vi "Approach then CV VUW.vi"(7 "Computer called (T/F)":bool) -> ()   [LabVIEW 2023]
uses:
  Sub_Vi/TypeDefsControls/Zposition.ctl
  Sub_Vi/TypeDefsControls/Piezo Velocity.ctl
  Sub_Vi/TypeDefsControls/Voltage.ctl
  Sub_Vi/TypeDefsControls/Xposition.ctl
  Sub_Vi/TypeDefsControls/Yposition.ctl
  Sub_Vi/TypeDefsControls/Voltage Scan Rate.ctl
  Sub_Vi/TypeDefsControls/Iterator.ctl
  Sub_Vi/TypeDefs/WayPointCluster.ctl
  Sub_Vi/TypeDefs/ChangeOnFly.ctl
  Sub_Vi/TypeDefs/Settings.ctl
  Sub_Vi/TypeDefs/Display.ctl
  Sub_Vi/TypeDefsControls/Feedback Type.ctl
  Settings.vi
panel:
  in  "Approach Type":u16=2
  out "Current 1":cluster{"Y":dbl[], "Y":dbl[]}[](graph)
  in  "Boolean Negative":bool
  in  "Boolean Positive":bool=TRUE
  in  "Feedback Threshold (A)\nGreater Than":dbl
  in  "Feedback Type":T1=enum."Current 1"
  in  "Display Cluster":T2
  in  "SettingsCluster":T3={"Sample Rate (us)"=1, "Samples Per Data Point (int, power of 2)"=1000, "DistanceToBulk (um)"=-1.0, "HoldTimeScaler"=1, "SaveData"=TRUE, "DistanceToBulk (um) 2"=-1.0, "DistanceToBulk (um) 3"=-1.0}
  in  "ChangeonFly":T4
  in  "WayPointCluster":T5
  in  "Number of Cycles":T6=1.0 min=1.0
  in  "Start scan Button":bool
  in  "Stop":bool
  in  "Pause":bool
  in  "Feedback Threshold (A)\nLess Than":dbl
  in  "Scan Rate (V/s)":T7 min=0.0 max=1000.0
  in  "Second Voltage (V)":T8 min=-10.0 max=10.0
  in  "First Voltage (V)":T8 min=-10.0 max=10.0
  in  "Set X":bool
  in  "Set Y":bool
  in  "Y":T9=100.0 min=0.0 max=100000.0
  in  "X":T10=100.0 min=0.0 max=100000.0
  in  "Approach Voltage (V)":T8 min=-10.0 max=10.0
  in  "Approach Rate (µm/s)":T11=0.1 min=0.0
  in  "End Extension (µm)":T12 min=0.0 max=100000.0
  in  "Start Extention (µm)":T12=150.0 min=0.0 max=100000.0
  out "?":cluster{"Y":dbl[], "Y":dbl[]}[](graph)
  out "?":dbl[](graph)
  # "Settings"
  # "Pause at"
  # "Advanced Settings"
  # "CV Controls"
  # "Voltage Profile"
  # "Approach"
  # "First Cycle"
  # "Additional Cycles"
  # "Retract"
  # "First\nVoltage"
  # "Approach\nVoltage"
  # "(Number of \ncycles)"
  # "Second\nVoltage"
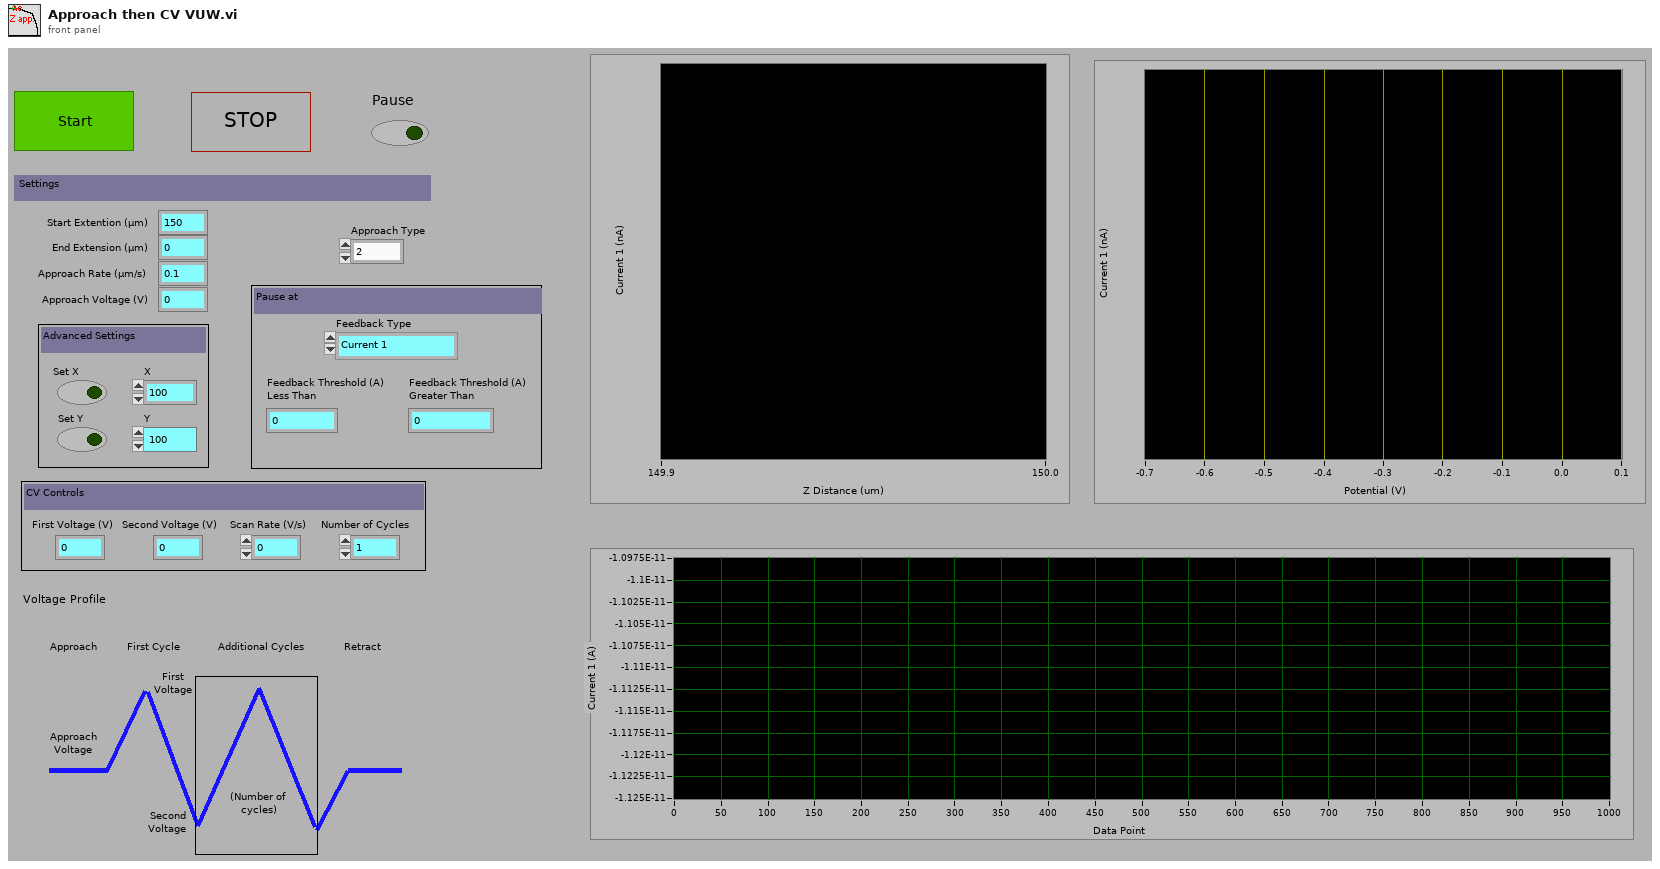
[diagram p1: front panel]
types:
  T1 = typedef "Feedback Type.ctl" = enum16{"AC Magnitude", "Current 1", "Current 2", "Phase"}
  T2 = typedef "Display.ctl" = cluster{"X":refnum<vi>, "Y":refnum<vi>, "Z":refnum<vi>, "Amp":refnum<vi>, "Phase":refnum<vi>, "t vs Z":refnum<vi>, "t vs C1":refnum<vi>, "t vs C2":refnum<vi>, "t vs C3":refnum<vi>, "t vs Amp":refnum<vi>, "t vs Phase":refnum<vi>, "t vs X":refnum<vi>, "t vs Y":refnum<vi>, "Z vs C1":refnum<vi>, "Z vs C2":refnum<vi>, "Z vs C3":refnum<vi>, "V vs C1":refnum<vi>, "V vs C2":refnum<vi>, "V vs C3":refnum<vi>, "X/Y/Z F":refnum<vi>, "X/Y/Z R":refnum<vi>, "X/Y/C1 F":refnum<vi>, "X/Y/C1 R":refnum<vi>, "X/Y/C2 F":refnum<vi>, "X/Y/C2 R":refnum<vi>, "X/Y/C3 F":refnum<vi>, "X/Y/C3 R":refnum<vi>, "NumberOfLines":u16, "um Per Pixel":dbl, "um Per Line":dbl, "X Center":dbl, "Hop X/Y/Z":refnum<vi>, "Hop X/Y/C1":refnum<vi>, "Hop X/Y/C2":refnum<vi>, "Hop X/Y/C3":refnum<vi>, "X Width":dbl, "Y Width":dbl, "Hopping Distance":dbl, "V2 vs C1":refnum<vi>, "V vs Phase":refnum<vi>, "Y Center":dbl, "Number of Pixels":dbl, "V2 vs C2":refnum<vi>, "V2 vs C3":refnum<vi>, "V vs y":refnum<vi>, "V2 vs y":refnum<vi>, "Z vs Amp":refnum<vi>, "Z vs Phase":refnum<vi>}
  T3 = typedef "Settings.ctl" = cluster{"Sample Rate (us)":u32, "Samples Per Data Point (int, power of 2)":i16, "DistanceToBulk (um)":dbl, "HoldTimeScaler":u64, "SaveData":bool, "DistanceToBulk (um) 2":dbl, "DistanceToBulk (um) 3":dbl}
  T4 = typedef "ChangeOnFly.ctl" = cluster{"Stop (boolean)":refnum<vi>, "Pause (boolean)":refnum<vi>, "EndCurrentLine (boolean)":refnum<vi>, "max movement per update step (Interger, nm)":refnum<vi>, "P (float, arb)":refnum<vi>, "Feedback set point (double, Amps)":refnum<vi>, "Voltage (double, V)":refnum<vi>, "Feedback set point 2 (double, Amps)":refnum<vi>, "Stop on Greater Than 2? (boolean)":refnum<vi>, "Stop on Greater Than? (boolean)":refnum<vi>, "Voltage 2 (double, V)":refnum<vi>, "Feedback Type (enum)":refnum<vi>, "Feedback Type 2 (enum)":refnum<vi>}
  T5 = typedef "WayPointCluster.ctl" = cluster{"X (um)":dbl[], "Y (um)":dbl[], "Z (um)":dbl[], "V (V)":dbl[], "X Velocity (um s-1)":dbl[], "Y Velocity (um s-1)":dbl[], "Z Velocity (um s-1)":dbl[], "V Velocity (V s-1)":dbl[], "FeedBack Type (enum)":u16[], "Move X (boolean)":bool[], "Move Y (boolean)":bool[], "Move Z (boolean)":bool[], "Move V (boolean)":bool[], "Jump V (boolean)":bool[], "Hold (boolean)":bool[], "Hold Time":u32[], "V2 (V)":dbl[], "Move V2":bool[], "V2 Velocity (V s-1)":dbl[], "Jump V2 (boolean)":bool[], "Update z Position delta (ms)":i16[], "Hold Feedback1":bool[], "Move Z PicoMotor":bool[], " Z PicoMotor Direction":bool[], "DIO0":bool[]}
  T6 = typedef "Iterator.ctl" = dbl
  T7 = typedef "Voltage Scan Rate.ctl" = dbl
  T8 = typedef "Voltage.ctl" = dbl
  T9 = typedef "Yposition.ctl" = dbl
  T10 = typedef "Xposition.ctl" = dbl
  T11 = typedef "Piezo Velocity.ctl" = dbl
  T12 = typedef "Zposition.ctl" = dbl
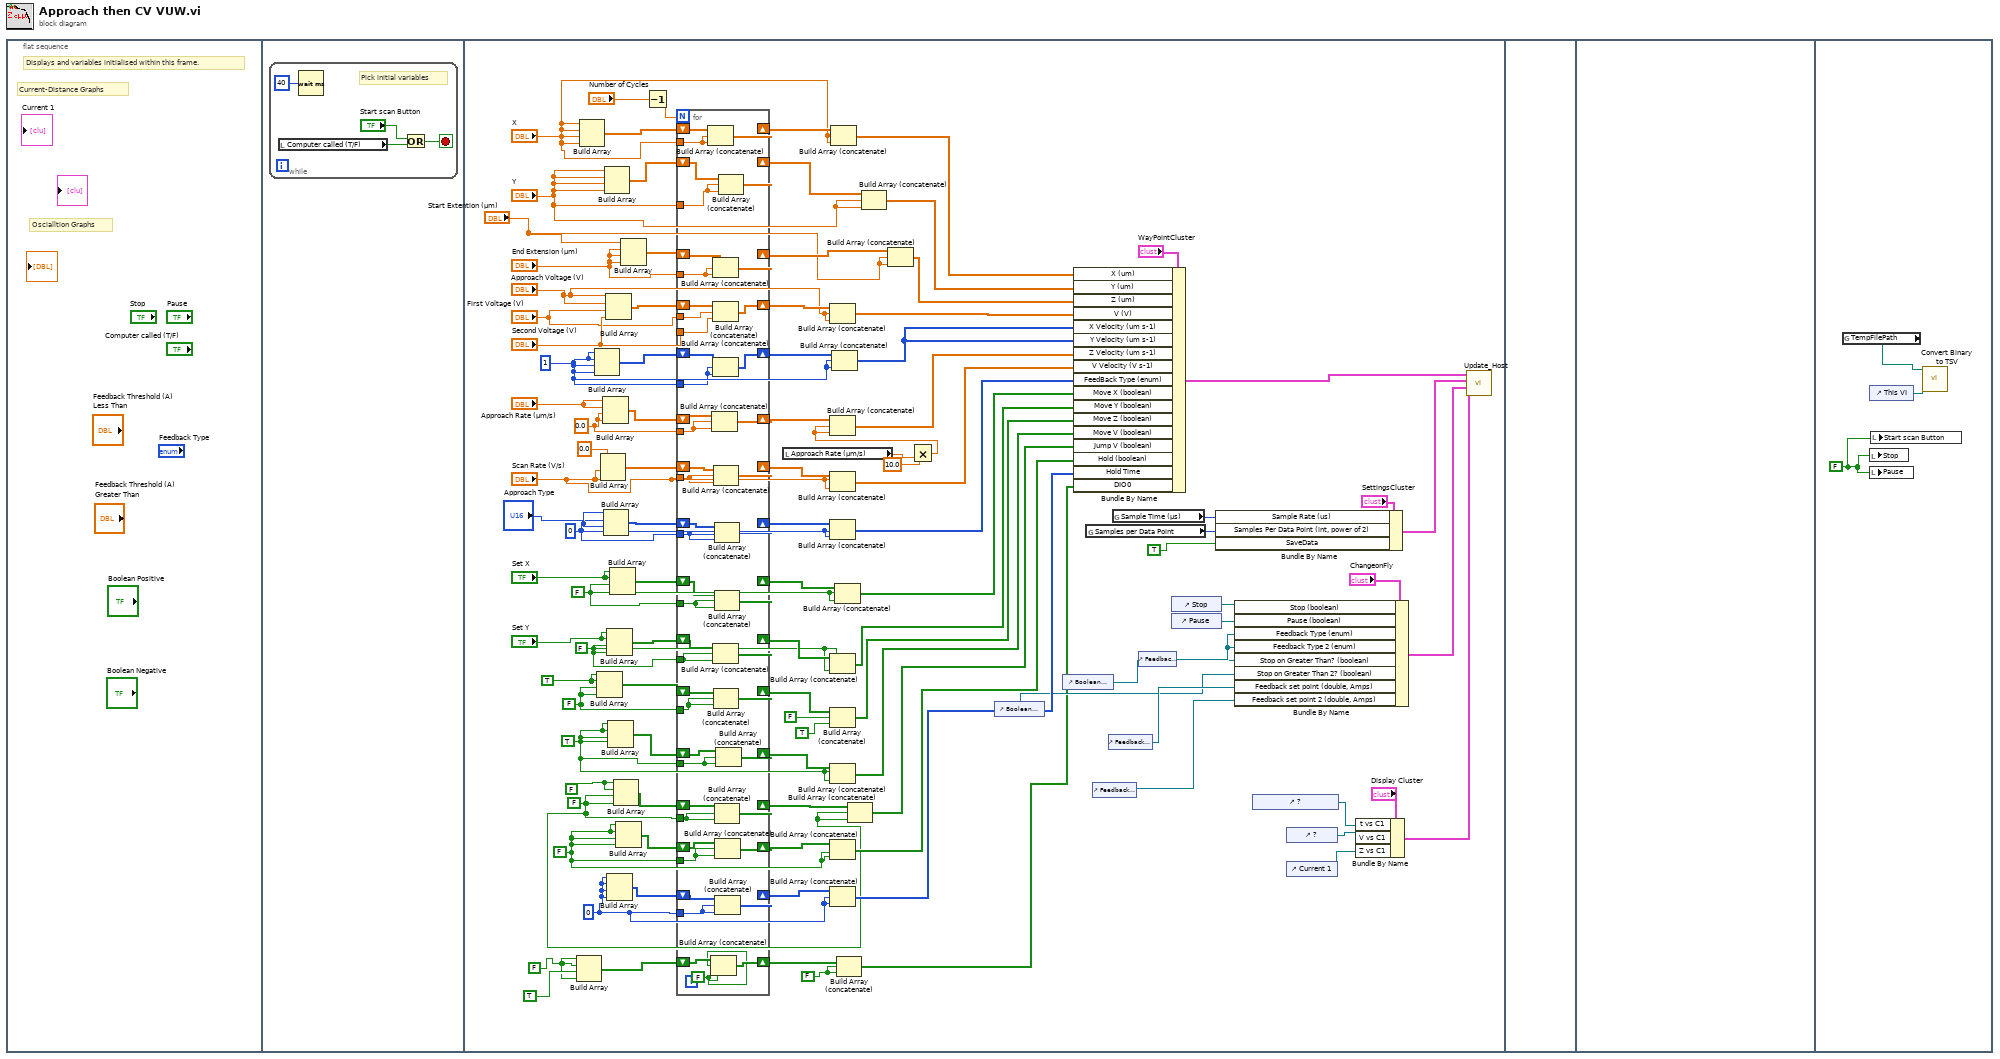
[diagram p0: block diagram]
diagram:
  n1 = flat-sequence {
    frame #0 {
      # "Oscialltion Graphs"
      # "Current-Distance Graphs"
      # "Displays and variables initialised within this frame."
    }
    frame #1 {
      n2 = while {
        stop <- w4 stop-if-true
        # "Pick initial variables"
        n3 = local read "Computer called (T/F)"() -> (w2:bool)
        n4 = Wait (ms)(milliseconds to wait=u32 40) -> ()  [unwired: 1 out]
        n5 = Or(x="Start scan Button", y=w2) -> (x .or. y?=w4:bool)
      }
    }
    frame #2 {
      w12 = FALSE ("Set Z")
      w6 = FALSE ("Set Z")
      w25 = u32 0 ("element")
      w9 = FALSE ("element")
      w8 = FALSE ("Set Z")
      w27 = TRUE ("element")
      w89 = FALSE ("element")
      w29 = FALSE ("element")
      w28 = FALSE ("element")
      w30 = u16 0 ("element")
      w54 = 0.0
      w34 = 0.0 ("element")
      w26 = FALSE ("Set Z")
      w51 = TRUE ("Set Z")
      w35 = 1
      n6 = Build Array(w6, w6, TRUE ("Set Z"), w6) -> (w14:bool[])
      n7 = Build Array("X", "X", "X", "X") -> (w59:T10[])
      n8 = Build Array(w35, w35, w35, w35) -> (w74:i32[])
      n9 = Build Array(w51, w51, w89, w89) -> (w90:bool[])
      n10 = Build Array(w54, w54, "Scan Rate (V/s)", "Scan Rate (V/s)") -> (w79:T7[])
      n11 = Build Array("Approach Rate (µm/s)", "Approach Rate (µm/s)", w34, w34) -> (w77:T11[])
      n12 = Build Array(w30, "Approach Type", w30, w30) -> (w82:u16[])
      n13 = Build Array("Y", "Y", "Y", "Y") -> (w62:T9[])
      n14 = Build Array("Approach Voltage (V)", "Approach Voltage (V)", "First Voltage (V)", "Second Voltage (V)") -> (w101:T8[])
      n15 = Build Array("Set Y", "Set Y", w28, w28) -> (w87:bool[])
      n16 = Build Array(w25, w25, w25, w25) -> (w100:u32[])
      n17 = Build Array(w27, w27, w27, w27) -> (w92:bool[])
      n18 = Build Array("Set X", "Set X", w29, w29) -> (w85:bool[])
      n19 = Build Array(w8, w8, w9, w9) -> (w94:bool[])
      n20 = Build Array(w26, w26, w26, w26) -> (w97:bool[])
      n21 = Build Array("Start Extention (µm)", "End Extension (µm)", "End Extension (µm)", "End Extension (µm)") -> (w41:T12[])
      n22 = Decrement(x="Number of Cycles") -> (x-1=w40:T6)
      n23 = for {
        N: w40 -> [_]
        tunnel: "First Voltage (V)" -> [w155]
        shift-right: [w156] -> w103
        shift-left: w101 -> [w157]
        tunnel: "Second Voltage (V)" -> [w154]
        shift-right: [w152] -> w99
        shift-left: w100 -> [w153]
        tunnel: w25 -> [w151]
        shift-right: [w148] -> w96
        shift-left: w97 -> [w149]
        tunnel: w26 -> [w150]
        shift-right: [w145] -> w93
        shift-left: w94 -> [w147]
        tunnel: w9 -> [w146]
        shift-right: [w143] -> w83
        shift-left: w92 -> [w144]
        tunnel: w27 -> [w142]
        shift-right: [w140] -> w91
        shift-left: w90 -> [w141]
        tunnel: w89 -> [w139]
        shift-right: [w137] -> w88
        shift-left: w87 -> [w138]
        tunnel: w28 -> [w136]
        shift-right: [w135] -> w84
        shift-left: w85 -> [w134]
        tunnel: w29 -> [w133]
        shift-right: [w131] -> w81
        shift-left: w82 -> [w132]
        tunnel: w30 -> [w130]
        shift-right: [w128] -> w80
        shift-left: w79 -> [w129]
        tunnel: "Scan Rate (V/s)" -> [w127]
        shift-right: [w125] -> w78
        shift-left: w77 -> [w126]
        tunnel: w34 -> [w124]
        shift-right: [w122] -> w75
        shift-left: w74 -> [w123]
        tunnel: w35 -> [w121]
        shift-right: [w120] -> w66
        shift-left: w41 -> [w119]
        tunnel: "End Extension (µm)" -> [w118]
        shift-right: [w116] -> w63
        shift-left: w62 -> [w117]
        tunnel: "Y" -> [w115]
        shift-right: [w113] -> w60
        shift-left: w59 -> [w114]
        tunnel: "X" -> [w112]
        shift-right: [w110] -> w13
        shift-left: w14 -> [w111]
        w109 = FALSE ("Set Z")
        n24 = Build Array (concatenate)(w114, w112, w112) -> (w113:T10[])
        n25 = Build Array (concatenate)(w111, w109, w109) -> (w110:bool[])
        n26 = Build Array (concatenate)(w126, w124, w124) -> (w125:T11[])
        n27 = Build Array (concatenate)(w119, w118, w118) -> (w120:T12[])
        n28 = Build Array (concatenate)(w157, w155, w154) -> (w156:T8[])
        n29 = Build Array (concatenate)(w123, w121, w121) -> (w122:i32[])
        n30 = Build Array (concatenate)(w138, w136, w136) -> (w137:bool[])
        n31 = Build Array (concatenate)(w129, w127, w127) -> (w128:T7[])
        n32 = Build Array (concatenate)(w141, w139, w139) -> (w140:bool[])
        n33 = Build Array (concatenate)(w132, w130, w130) -> (w131:u16[])
        n34 = Build Array (concatenate)(w134, w133, w133) -> (w135:bool[])
        n35 = Build Array (concatenate)(w147, w146, w146) -> (w145:bool[])
        n36 = Build Array (concatenate)(w149, w150, w150) -> (w148:bool[])
        n37 = Build Array (concatenate)(w153, w151, w151) -> (w152:u32[])
        n38 = Build Array (concatenate)(w144, w142, w142) -> (w143:bool[])
        n39 = Build Array (concatenate)(w117, w115, w115) -> (w116:T9[])
      }
      n40 = local read "Approach Rate (µm/s)"() -> (w33:T11)
      n41 = Build Array (concatenate)(w103, "Approach Voltage (V)", "Approach Voltage (V)") -> (w102:T8[])
      n42 = Build Array (concatenate)(w80, "Scan Rate (V/s)", "Scan Rate (V/s)") -> (w67:T7[])
      n43 = Build Array (concatenate)(w81, w30, w30) -> (w68:u16[])
      n44 = Build Array (concatenate)(w88, w28, w28) -> (w69:bool[])
      n45 = Build Array (concatenate)(w91, FALSE ("Set Z"), TRUE ("Set Z")) -> (w70:bool[])
      n46 = Build Array (concatenate)(w83, w27, w27) -> (w71:bool[])
      n47 = Build Array (concatenate)(w96, w26, w26) -> (w95:bool[])
      n48 = Build Array (concatenate)(w99, w25, w25) -> (w98:u32[])
      n49 = Build Array (concatenate)(w60, "X", "X") -> (w58:T10[])
      n50 = Build Array (concatenate)(w75, w35, w35) -> (w73:i32[])
      n51 = Build Array (concatenate)(w84, w29, w29) -> (w86:bool[])
      n52 = Build Array (concatenate)(w13, w12, w12) -> (w11:bool[])
      n53 = Build Array (concatenate)(w93, w9, w9) -> (w72:bool[])
      n54 = Build Array (concatenate)(w63, "Y", "Y") -> (w61:T9[])
      n55 = Build Array (concatenate)(w66, "Start Extention (µm)", "Start Extention (µm)") -> (w64:T12[])
      n56 = Multiply(x=T11 10.0, y=w33) -> (x*y=w18:T11)
      n57 = Build Array (concatenate)(w78, w18, w18) -> (w76:T11[])
      n58 = control-ref of="Boolean Negative"() -> (w20:refnum<vi>)
      n59 = control-ref of="Boolean Positive"() -> (w21:refnum<vi>)
      n60 = Bundle By Name(cluster="WayPointCluster", "X (um)"=w58, "Y (um)"=w61, "Z (um)"=w64, "V (V)"=w102, "X Velocity (um s-1)"=w73, "Y Velocity (um s-1)"=w73, "Z Velocity (um s-1)"=w76, "V Velocity (V s-1)"=w67, "FeedBack Type (enum)"=w68, "Move X (boolean)"=w86, "Move Y (boolean)"=w69, "Move Z (boolean)"=w70, "Move V (boolean)"=w71, "Jump V (boolean)"=w72, "Hold (boolean)"=w95, "Hold Time"=w98, "DIO0"=w11) -> (w108:T5)
      n61 = global read "Settings.vi" "Samples per Data Point"() -> (w47:u16)
      n62 = control-ref of="Feedback Threshold (A)\nGreater Than"() -> (w22:refnum<vi>)
      n63 = control-ref of="Feedback Threshold (A)\nLess Than"() -> (w23:refnum<vi>)
      n64 = global read "Settings.vi" "Sample Time (µs)"() -> (w48:u32)
      n65 = control-ref of="Feedback Type"() -> (w24:refnum<vi>)
      n66 = control-ref of="Stop"() -> (w104:refnum<vi>)
      n67 = control-ref of="Pause"() -> (w5:refnum<vi>)
      n68 = Bundle By Name(cluster="SettingsCluster", "Sample Rate (us)"=w48, "Samples Per Data Point (int, power of 2)"=w47, "SaveData"=TRUE) -> (w106:T3)
      n69 = Bundle By Name(cluster="ChangeonFly", "Stop (boolean)"=w104, "Pause (boolean)"=w5, "Feedback Type (enum)"=w24, "Feedback Type 2 (enum)"=w24, "Stop on Greater Than? (boolean)"=w21, "Stop on Greater Than 2? (boolean)"=w20, "Feedback set point (double, Amps)"=w23, "Feedback set point 2 (double, Amps)"=w22) -> (w105:T4)
      n70 = control-ref of="?"() -> (w19:refnum<vi>)
      n71 = control-ref of="?"() -> (w45:refnum<vi>)
      n72 = control-ref of="Current 1"() -> (w44:refnum<vi>)
      n73 = Bundle By Name(cluster="Display Cluster", "t vs C1"=w19, "V vs C1"=w45, "Z vs C1"=w44) -> (w107:T2)
      n74 = call "Update_Host.vi"("Display Cluster"=w107, "ChangeonFly"=w105, "SettingsCluster"=w106, "WayPointCluster"=w108) -> ()  [unwired: 6 in]
    }
    frame #3 {
    }
    frame #4 {
    }
    frame #5 {
      w159 = FALSE ("Start Scanning Button")
      n75 = global read "Settings.vi" "TempFilePath"() -> (w158:path)
      n76 = control-ref of="This VI"() -> (w160:refnum<vi>)
      n77 = local write "Stop"(w159) -> ()
      n78 = local write "Pause"(w159) -> ()
      n79 = local write "Start scan Button"(w159) -> ()
      n80 = call "Convert Binary to TSV.vi"("This VI"=w160, "TDMS DataFile Name"=w158) -> ()  [unwired: 10 in]
    }
  }
